vi "WriteCmdOut.vi"(0 "Connections In":T1(array[cluster]), 2 "Log in":T2[](array[typedef]), 3 "Err in":path, 4 "data":string) -> (5 "Connections Out":T1(array[cluster]), 6 "Log out":T2[](array[typedef]), 7 "Err out":path)   [LabVIEW 2012]
uses:
  <userlib>/ROSforLV/ROS/Code/Console/Servers/ServerSubs/ROSLog.ctl
  <userlib>/ROSforLV/ROS/Code/_ROSDefinition.vi
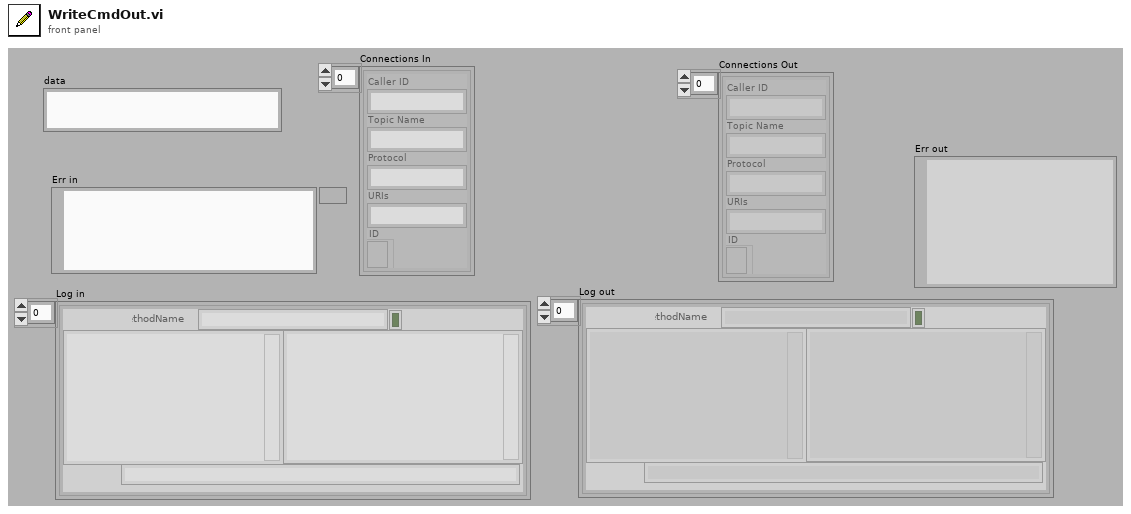
[diagram p1: front panel]
types:
  T1 = cluster{"Caller ID":string, "Topic Name":string, "Protocol":string, "URIs":string, "ID":refnum<k5>}[]
  T2 = typedef "ROSLog.ctl" = cluster{"Sent":string, "Reply":string, "MethodName":string, "success":bool, "Dir1":string, "Dir2":string, "Time Stamp":string, "error":errorcluster, "Preamble":string}
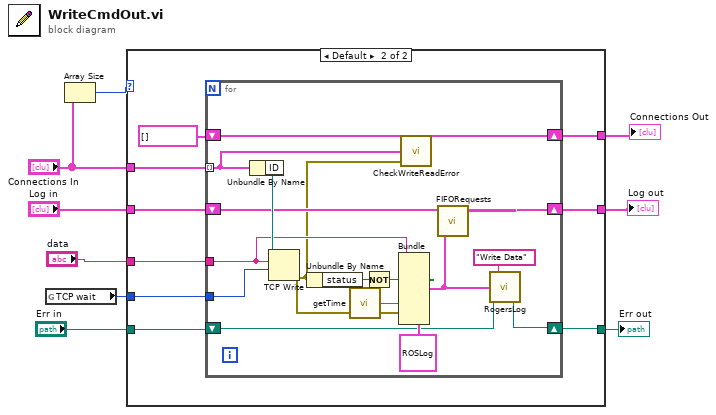
[diagram p0: block diagram]
diagram:
  n1 = global read "_ROSDefinition.vi" "TCP wait"() -> (w1:i32)
  n2 = Array Size(array="Connections In") -> (size(s)=w4:i32)
  n3 = case shown="Default" w4 {
    tunnel: [w12 w21] -> w9
    tunnel: "Log in" -> [w12 w20]
    tunnel: "Err in" -> [w11 w19]
    tunnel: [w11 w18] -> w6
    tunnel: "Connections In" -> [w10 w17]
    tunnel: "data" -> [_ w16]
    tunnel: [w10 w14] -> w2
    tunnel: w1 -> [_ w13]
    frame 0 {
    }
    frame Default {
      n4 = for {
        shift-right: [w24] -> w18
        shift-left: w19 -> [w25]
        shift-right: [w32] -> w21
        shift-left: w20 -> [w33]
        tunnel: w17 -> [w31] mode=indexing
        tunnel: w16 -> [w34]
        shift-right: [w29] -> w14
        shift-left: T1 [] -> [w28]
        tunnel: w13 -> [w27]
        n5 = Unbundle By Name(w31) -> ("ID"=w38:refnum<k5>)
        n6 = TCP Write(connection ID=w38, data in=w34, 9:w27) -> (error out=w26:errorcluster)  [unwired: 1 in, 2 out]
        n7 = Unbundle By Name(w26) -> ("status"=w36:bool)
        n8 = call <userlib>:"getTime.vi"() -> ("Current Time"=w37:string)  [unwired: 1 in]
        n9 = Not(x=w36) -> (.not. x?=w35:bool)
        n10 = Bundle(cluster=T2 {"Sent"="", "Reply"="", "MethodName"="write", "success"=FALSE, "Dir1"="To ROS", "Dir2"="From ROS", "Time Stamp"="", "error"={"status"=FALSE, "code"=0, "source"=""}, "Preamble"=""} ("Log"), "Sent"=w34, "success"=w35, "Time Stamp"=w37, "error"=w26) -> (w23:T2)  [unwired: 5 in]
        n11 = call <userlib>:"CheckWriteReadError.vi"("error"=w26, "Subscriber in"=w31, "Connections in"=w28) -> ("Connections out"=w29:T1)
        n12 = call <userlib>:"FIFORequests.vi"("Log"=w23, "Requests in"=w33) -> ("Requests out"=w32:T2[])  [unwired: 1 in]
        n13 = call <userlib>:"RogersLog.vi"("Text to add"="Write Data", "Log"=w23, "LogPath in"=w25) -> ("LogPath out"=w24:path)  [unwired: 2 in, 1 out]
      }
    }
  }
  "Log out" <- w9
  "Err out" <- w6
  "Connections Out" <- w2
